vi "_Serial_Mark10-Connection_Check.vi"(5 "Serial Port":refnum<visa-resource-name>="COM5") -> (1 "Normal reception":bool, 2 "VISA resource name out":refnum<visa-resource-name>)   [LabVIEW 2015]
uses:
  <vilib>/Instr/_visa.llb/VISA Configure Serial Port (Instr).vi
panel:
  out "Read Buffer":string
  out "Port Connection Normal":bool
  # "MARK10 Connection State Checking"
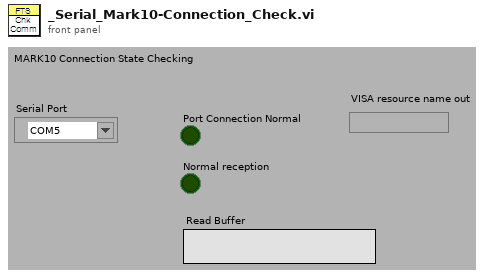
[diagram p1: front panel]
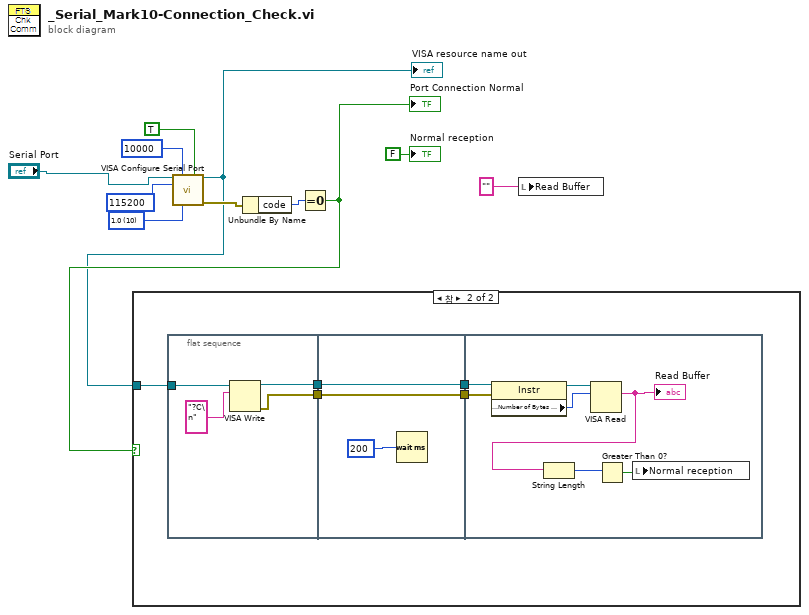
[diagram p0: block diagram]
diagram:
  w8 = u16 10 items=["1.0"=10, "1.5"=15, "2.0"=20] ("stop bits (10: 1 bit)")
  n1 = call-poly "VISA Configure Serial Port"("VISA resource name"="Serial Port", "timeout (10sec)"=u32 10000, "Enable Termination\nChar (T)"=TRUE ("Enable Termination\nChar (T)"), "baud rate (9600)"=u32 115200, "stop bits (10: 1 bit)"=w8) -> ("VISA resource name out"=w3:refnum<visa-resource-name>, "error out"=w10:errorcluster)  [unwired: 4 in, 5 out]
  "VISA resource name out" <- w3
  n2 = Unbundle By Name(w10) -> ("code"=w9:i32)
  n3 = Equal To 0?(x=w9) -> (x = 0?=w4:bool)
  "Port Connection Normal" <- w4
  n4 = case shown="참" w4 {
    tunnel: w3 -> [_ w16]
    frame False {
    }
    frame True {
      n5 = flat-sequence {
        tunnel: w16 -> [w20]
        tunnel: [w18] -> w15
        tunnel: [w17] -> w12
        tunnel: w15 -> [w22]
        tunnel: [w22] -> w14
        tunnel: [w21] -> w13
        tunnel: w12 -> [w21]
        tunnel: w14 -> [w28]
        tunnel: w13 -> [w27]
        frame #0 {
          n6 = VISA Write(VISA resource name=w20, write buffer="?C\n") -> (VISA resource name out=w18:refnum<visa-resource-name>, error out=w17:errorcluster)  [unwired: 1 in, 1 out]
        }
        frame #1 {
          n7 = Wait (ms)(milliseconds to wait=u32 200 ("대기 시간(ms)")) -> ()  [unwired: 1 out]
        }
        frame #2 {
          n8 = property class="Instr"(reference=w28, error in=w27) -> (reference out=w29:refnum<visa-resource-name>, "Serial Settings:Number of Bytes at Serial Port"=w30:u32)  [unwired: 1 out]
          n9 = VISA Read(VISA resource name=w29, byte count=w30) -> (read buffer=w26:string)  [unwired: 1 in, 3 out]
          "Read Buffer" <- w26
          n10 = String Length(string=w26) -> (length=w25:i32)
          n11 = Greater Than 0?(x=w25) -> (x > 0?=w24:bool)
          n12 = local write "Normal reception"(w24) -> ()
        }
      }
    }
  }
  n13 = local write "Read Buffer"("" ("버퍼 읽기")) -> ()
  "Normal reception" <- FALSE ("수신 정상")
